vi "getTimeSinceEpoch.vi"(1 "TLE":string, 2 "UTC":dbl) -> (0 "number of minutes since\nthe epoch (t-t0) (min)":dbl format="%#_13g")   [LabVIEW 2015]
uses:
  <vilib>/imath/engines/lvmath2/RunTimeEngine/BuiltInFunctions/mod/NIMS_mod_no_size_check.vi
  <instcachedir>/0/NIMS_mod_no_size_check_5393E3382FD241D281EEB71DA286C65B.lvgen/NIMS_mod_no_size_check_5393E3382FD241D281EEB71DA286C65B_001.vi
  <vilib>/imath/engines/lvmath2/RunTimeEngine/NodeEndStatement/NIMS_NodeEndStatement_Output.vi
  <instcachedir>/0/NIMS_NodeEndStatement_Output_53EC0D466D134D7ABD903AC30B43404B.lvgen/NIMS_NodeEndStatement_Output_53EC0D466D134D7ABD903AC30B43404B_012.vi
  <vilib>/imath/engines/lvmath2/RunTimeEngine/ErrorHandling/NIMS_Finalize Error.vi
panel:
  out "TLE year":dbl format="%#_13g"
  out "number of seconds since the \nJanuary 1st 1904":dbl format="%#_13g"
  out "number of minutes \nof the epoch (min)":i32
  out "fraction of the day":dbl format="%#_13g"
  out "number of the day during the \nyear where the TLE has been determined":dbl format="%#_13g"
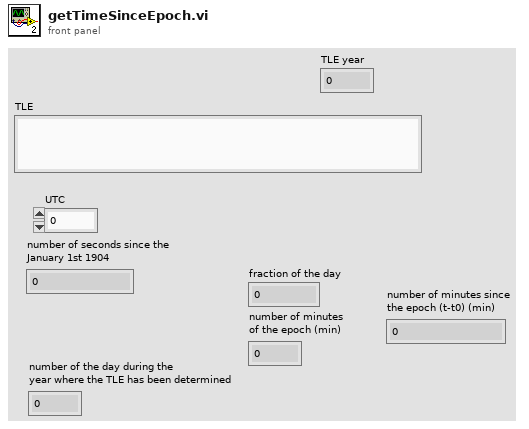
[diagram p1: front panel]
types:
  T1 = cluster{"second":i32, "minute":i32, "hour":i32, "day of month":i32, "month":i32, "year":i32, "day of week":i32, "day of year":i32, "is DST":i32}
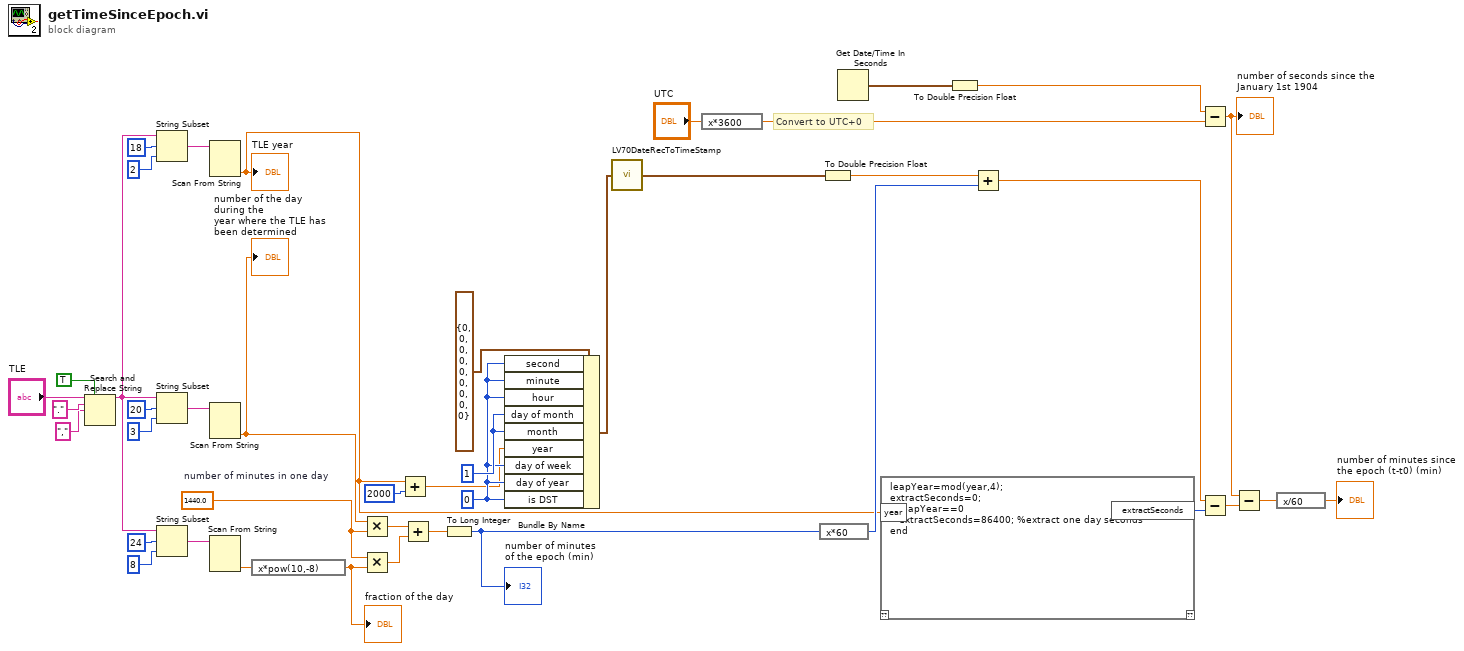
[diagram p0: block diagram]
diagram:
  w17 = 1
  w16 = 0
  w30 = 1440.0  # number of minutes in one day
  # "Convert to UTC+0"
  n1 = Search and Replace String(replace all?=TRUE, input string="TLE", search string=".", replace string=",") -> (result string=w21:string)  [unwired: 4 in, 3 out]
  n2 = String Subset(string=w21, offset (0)=18, length (rest)=2) -> (substring=w20:string)
  n3 = String Subset(string=w21, offset (0)=20, length (rest)=3) -> (substring=w36:string)
  n4 = String Subset(string=w21, offset (0)=24, length (rest)=8) -> (substring=w33:string)
  n5 = Scan From String(input string=w20) -> (output 1=w4:dbl)  [unwired: 4 in, 3 out]
  "TLE year" <- w4
  n6 = Scan From String(input string=w36) -> (output 1=w7:dbl)  [unwired: 4 in, 3 out]
  "number of the day during the \nyear where the TLE has been determined" <- w7
  n7 = Scan From String(input string=w33) -> (output 1=w32:dbl)  [unwired: 4 in, 3 out]
  n8 = expression code="x*pow(10,-8)"(w32) -> (w31:dbl)
  "fraction of the day" <- w31
  n9 = Multiply(x=w7, y=w30) -> (x*y=w6:dbl)
  n10 = Multiply(x=w30, y=w31) -> (x*y=w29:dbl)
  n11 = Add(x=w4, y=2000) -> (x+y=w14:dbl)
  n12 = Add(x=w6, y=w29) -> (x+y=w28:dbl)
  n13 = To Long Integer(number=w28) -> (32bit integer=w25:i32)
  "number of minutes \nof the epoch (min)" <- w25
  n14 = Bundle By Name(cluster=T1 {"second"=0, "minute"=0, "hour"=0, "day of month"=0, "month"=0, "year"=0, "day of week"=0, "day of year"=0, "is DST"=0} ("date time rec"), "second"=w16, "minute"=w16, "hour"=w16, "day of month"=w17, "month"=w17, "year"=w14, "day of week"=w16, "day of year"=w16, "is DST"=w16) -> (w18:T1)
  n15 = call <vilib>:"LV70DateRecToTimeStamp.vi"("date time rec"=w18) -> ("Time Stamp"=w13:timestamp)
  n16 = expression code="x*3600"("UTC") -> (w9:dbl)
  n17 = expression code="x*60"(w25) -> (w12:i32)
  n18 = To Double Precision Float(number=w13) -> (double precision float=w5:dbl)
  n19 = Get Date/Time In Seconds() -> (seconds since 1Jan1904=w27:timestamp)
  n20 = mathscript code="leapYear=mod(year,4);\nextractSeconds=0;\nif leapYear==0\n   extractSeconds=86400; %extract one day seconds\nend"("year"=w4) -> ("extractSeconds"=w2:i32)  [unwired: 1 in, 1 out]
  n21 = To Double Precision Float(number=w27) -> (double precision float=w10:dbl)
  n22 = Add(x=w5, y=w12) -> (x+y=w3:dbl)
  n23 = Subtract(x=w10, y=w9) -> (x-y=w11:dbl)
  "number of seconds since the \nJanuary 1st 1904" <- w11
  n24 = Subtract(x=w3, y=w2) -> (x-y=w1:dbl)
  n25 = Subtract(x=w11, y=w1) -> (x-y=w26:dbl)
  n26 = expression code="x/60"(w26) -> (→"number of minutes since\nthe epoch (t-t0) (min)":dbl)
